vi "lookuptable.vi"(8 "array_y":dbl[](array[numeric]), 9 "array_x":dbl[](array[numeric]), 11 "x":dbl) -> (3 "y":dbl)   [LabVIEW 2015]
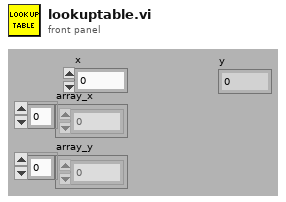
[diagram p1: front panel]
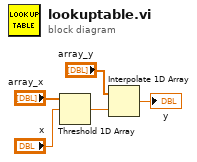
[diagram p0: block diagram]
diagram:
  n1 = Threshold 1D Array(2:"x", 3:"array_x") -> (0:w2:dbl)  [unwired: 1 in]
  n2 = Interpolate 1D Array(1:w2, 2:"array_y") -> (0:→"y":dbl)
